vi "IMAQ FPGA Image Transfer to Target U32.vi"(6 "Image Transfer Size Alignment":u32(ring)=1 items=["1 Pixel"=1, "8 Pixels"=8], 7 "Write Timeout (ms)":i32=5000, 8 "error in (no error)":errorcluster, 9 "DMA FIFO Reference In":refnum<k20>, 10 "Maximum Pixels per Write":i32=-1, 11 "Image":T1) -> (0 "error out":errorcluster, 1 "DMA FIFO Reference Out":refnum<k20>, 3 "Image Out":T1)   [LabVIEW 2020, in "NI_VDM_FPGA_Basics.lvlib"]
doc: "Transfers an image from the host processor to the target FPGA via a DMA FIFO."
uses:
  <vilib>/visionFPGA/NI_VDM_FPGA_Basics.lvlib
  <vilib>/vision/Image Controls.llb/IMAQ Image.ctl
  <vilib>/rvi/errors/niLvFpgaAdjustHostInterfaceError.vi
  <vilib>/rvi/interface/nirviMethod/nirviMethod.xnode
  <vilib>/rvi/errors/niLvFpgaMergeErrorWithErrorCode.vi
  nivissvc.dll
  <vilib>/FPGAPlugInAG/Dynamic/niLvFpga_AcquireWriteRegionFifo_Dynamic.vi
  <vilib>/FPGAPlugInAG/Dynamic/niLvFpga_WriteFifo_Dynamic.vi
  <vilib>/vision/EDVR.llb/IMAQ ImageToEDVR 2D U32.vi
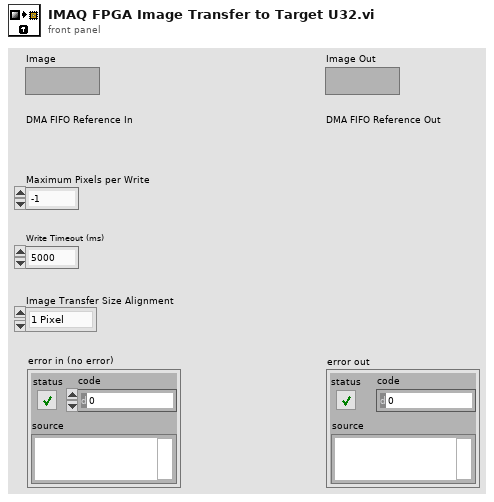
[diagram p1: front panel]
types:
  T1 = typedef "IMAQ Image.ctl" = refnum<image>
  T2 = typedef "Image Type" = u32
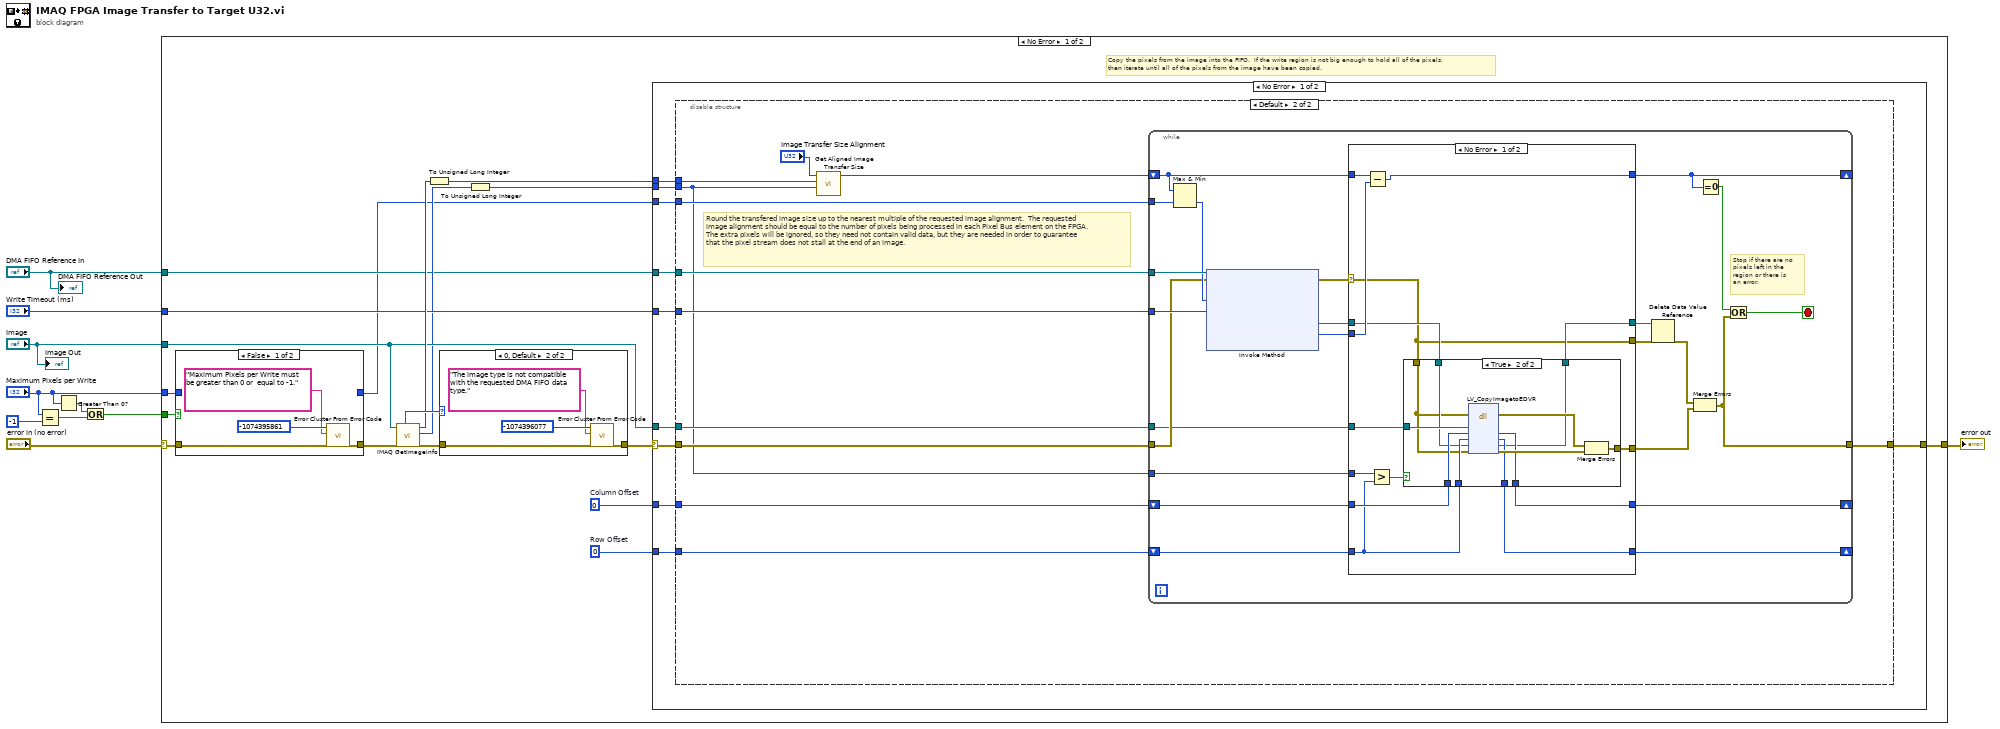
[diagram p0: block diagram]
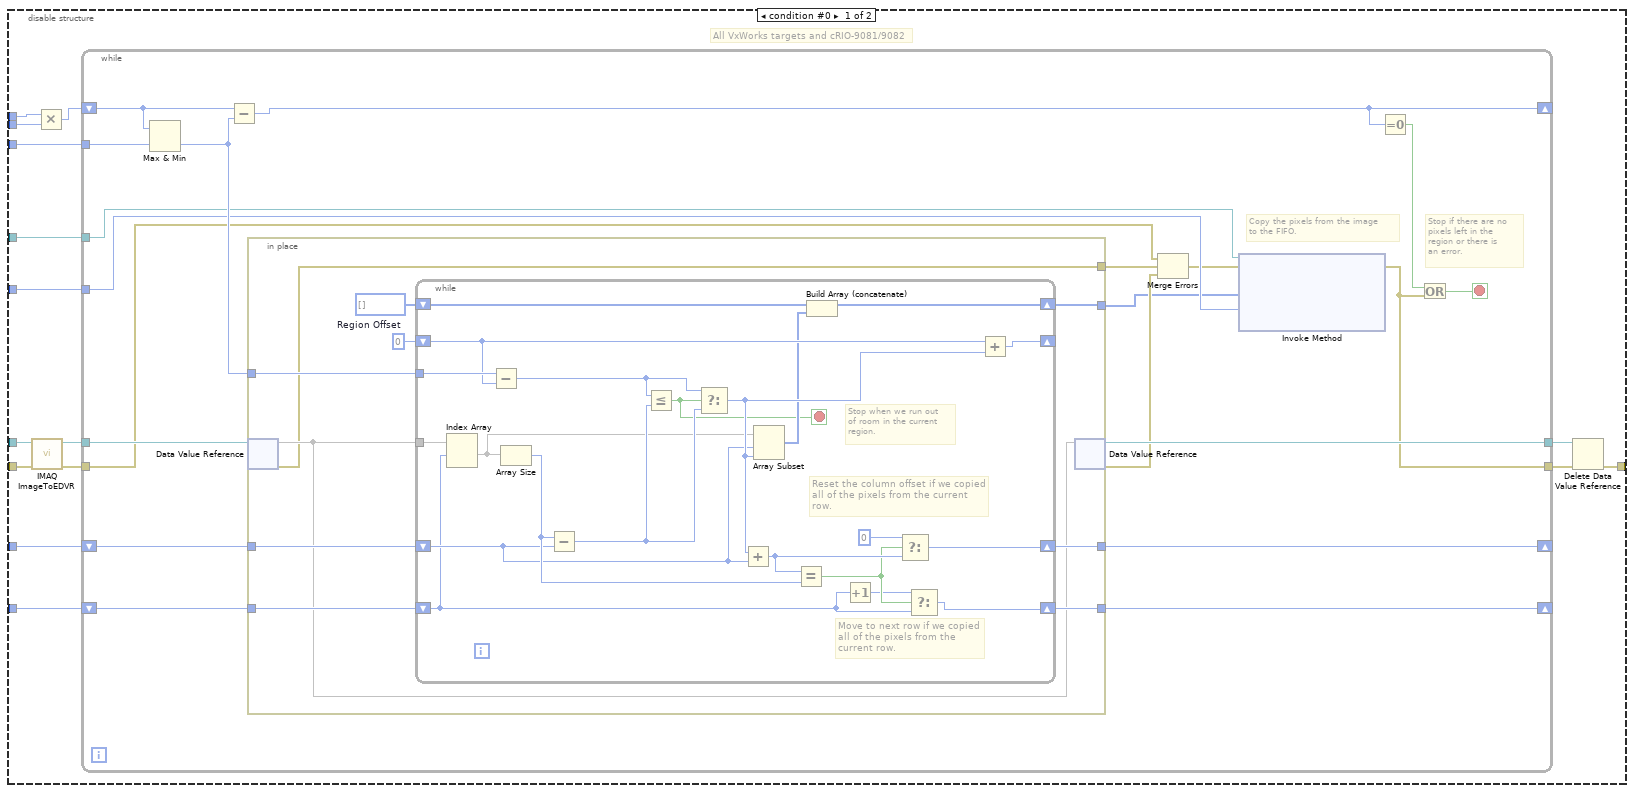
[diagram p2: hidden frame]
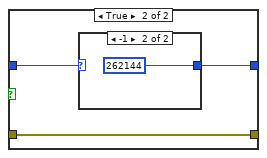
[diagram p6: hidden frame]
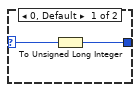
[diagram p7: hidden frame]
diagram:
  n1 = Equal?(x="Maximum Pixels per Write", y=-1) -> (x = y?=w6:bool)
  n2 = Greater Than 0?(x="Maximum Pixels per Write") -> (x > 0?=w7:bool)
  n3 = Or(x=w7, y=w6) -> (x .or. y?=w5:bool)
  n4 = case shown="No Error" "error in (no error)" {
    selector: "error in (no error)" -> [w23 w190]
    tunnel: "DMA FIFO Reference In" -> [w14 _]
    tunnel: "Write Timeout (ms)" -> [w16 _]
    tunnel: w5 -> [w26 _]
    tunnel: "Maximum Pixels per Write" -> [w24 _]
    tunnel: "Image" -> [w18 _]
    tunnel: [w21 w190] -> w2
    frame No Error {
      w20 = u32 0  # Row Offset
      w19 = u32 0  # Column Offset
      # "Copy the pixels from the image into the FIFO.  If the write region is not big enough to hold all of the pixels,\nthen iterate until all of the pixels from the image have been copied."
      n5 = case shown="False" w26 {
        tunnel: w23 -> [w176 w181]
        tunnel: [w175 w181] -> w25
        tunnel: w24 -> [_ w180]
        tunnel: [_ w179] -> w13
        frame False {
          n6 = call <vilib>:"Error Cluster From Error Code.vi"("error in (no error)"=w176, "error message (\"\")"="Maximum Pixels per Write must be greater than 0 or  equal to -1." ("error message (\"\")"), "error code (0)"=-1074395861) -> ("error out"=w175:errorcluster)  [unwired: 6 in]
        }
        frame True {
          n7 = case shown="-1" w180 {
            selector: w180 -> [w183 _]
            tunnel: [w182 u32 262144 ("Maximum Pixels per Write")] -> w179
            frame 0, Default {
              n8 = To Unsigned Long Integer(number=w183) -> (unsigned 32bit integer=w182:u32)
            }
            frame -1 {
            }
          }
        }
      }
      n9 = call "IMAQ GetImageInfo"("error in (no error)"=w25, "Image"=w18) -> ("error out"=w27:errorcluster, "Y Resolution"=w15:i32, "X Resolution"=w22:i32, "Image Type"=w28:T2)  [unwired: 2 in, 4 out]
      n10 = To Unsigned Long Integer(number=w22) -> (unsigned 32bit integer=w12:u32)
      n11 = case shown="0, Default" w28 {
        tunnel: w27 -> [w185 w187]
        tunnel: [w185 w186] -> w17
        frame 4, 5 {
          # "Allowed types are:\nRGB (U32)\nHSL (U32)"
        }
        frame 0, Default {
          n12 = call <vilib>:"Error Cluster From Error Code.vi"("error in (no error)"=w187, "error message (\"\")"="The image type is not compatible with the requested DMA FIFO data type." ("error message (\"\")"), "error code (0)"=-1074396077) -> ("error out"=w186:errorcluster)  [unwired: 6 in]
        }
      }
      n13 = To Unsigned Long Integer(number=w15) -> (unsigned 32bit integer=w11:u32)
      n14 = case shown="No Error" w17 {
        selector: w17 -> [w33 w174]
        tunnel: w19 -> [w35 _]
        tunnel: w20 -> [w34 _]
        tunnel: w14 -> [w37 _]
        tunnel: [w31 w174] -> w21
        tunnel: w13 -> [w38 _]
        tunnel: w16 -> [w36 _]
        tunnel: w18 -> [w32 _]
        tunnel: w12 -> [w30 _]
        tunnel: w11 -> [w29 _]
        frame No Error {
          n15 = disable-structure shown="Default" {
            disable-tunnel: w35 -> [w53 w116]
            disable-tunnel: w34 -> [w52 w115]
            disable-tunnel: w37 -> [w51 w114]
            disable-tunnel: [w42 w113] -> w31
            disable-tunnel: w38 -> [w50 w112]
            disable-tunnel: w36 -> [w49 w111]
            disable-tunnel: w33 -> [w47 w110]
            disable-tunnel: w32 -> [w48 w109]
            disable-tunnel: w30 -> [w40 w106]
            disable-tunnel: w29 -> [w41 w105]
            frame condition #0 {
              # "All VxWorks targets and cRIO-9081/9082"
              n16 = call-poly <vilib>:"IMAQ ImageToEDVR.vi"("error out"=w47, "Image"=w48) -> ("error out"=w45:errorcluster, "EDVR 2D U32"=w46:refnum<data-value>)  [unwired: 7 in, 1 out]
              n17 = Multiply(x=w40, y=w41) -> (x*y=w39:u32)
              n18 = while {
                shift-right: [w67] -> _
                shift-left: w39 -> [w64]
                tunnel: w46 -> [w73]
                shift-right: [w69] -> _
                shift-left: w53 -> [w71]
                shift-right: [w72] -> _
                shift-left: w52 -> [w70]
                tunnel: w51 -> [w58]
                tunnel: [w68] -> w44
                tunnel: [w56] -> w43
                tunnel: w50 -> [w63]
                tunnel: w49 -> [w59]
                tunnel: w45 -> [w54]
                stop <- w66 stop-if-true
                # "Copy the pixels from the image\nto the FIFO."
                # "Stop if there are no\npixels left in the \nregion or there is\nan error."
                n19 = Max & Min(x=w64, y=w63) -> (min(x,y)=w62:u32)  [unwired: 1 out]
                n20 = Subtract(x=w64, y=w62) -> (x-y=w67:u32)
                n21 = in-place {
                  in-place-border: w62 -> [w81]
                  in-place-border: [w83] -> w72
                  in-place-border: w71 -> [w80]
                  in-place-border: w70 -> [w78]
                  in-place-border: [w79] -> w69
                  in-place-border: [w75] -> w61
                  in-place-border: [w74] -> w55
                  w82 = u32 0  # Region Offset
                  n22 = in-place-dvr #1(w73) -> (w77:u32[][], w75:errorcluster)
                  n23 = while {
                    tunnel: w77 -> [w90]
                    shift-right: [w102] -> _
                    shift-left: w82 -> [w101]
                    tunnel: w81 -> [w104]
                    shift-right: [w95] -> w79
                    shift-left: w80 -> [w91]
                    shift-right: [w85] -> w74
                    shift-left: u8[] [] -> [w87]
                    shift-right: [w92] -> w83
                    shift-left: w78 -> [w88]
                    stop <- w84 stop-if-true
                    # "Stop when we run out\nof room in the current\nregion."
                    # "Reset the column offset if we copied\nall of the pixels from the current\nrow."
                    # "Move to next row if we copied\nall of the pixels from the\ncurrent row."
                    n24 = Index Array(array=w90, index (row)=w88) -> (element=w89:u32[])  [unwired: 1 in]
                    n25 = Subtract(x=w104, y=w101) -> (x-y=w103:u32)
                    n26 = Array Size(array=w89) -> (size(s)=w100:i32)
                    n27 = Subtract(x=w100, y=w91) -> (x-y=w98:u32)
                    n28 = Less Or Equal?(x=w103, y=w98) -> (x <= y?=w84:bool)
                    n29 = Select(t=w103, s=w84, f=w98) -> (s? t:f=w99:u32)
                    n30 = Add(x=w99, y=w91) -> (x+y=w96:u32)
                    n31 = Array Subset(array=w89, index=w91, length=w99) -> (w86:u32[])
                    n32 = Equal?(x=w96, y=w100) -> (x = y?=w94:bool)
                    n33 = Build Array (concatenate)(w87, w86) -> (w85:u32[])
                    n34 = Increment(x=w88) -> (x+1=w93:u32)
                    n35 = Select(t=u32 0 ("Elements In Region"), s=w94, f=w96) -> (s? t:f=w95:u32)
                    n36 = Select(t=w93, s=w94, f=w88) -> (s? t:f=w92:u32)
                    n37 = Add(x=w101, y=w99) -> (x+y=w102:u32)
                  }
                  n38 = in-place-dvr #1(w77) -> (w68:refnum<data-value>, w60:errorcluster)
                }
                n39 = Merge Errors(w54, w61, w60) -> (w57:errorcluster)
                n40 = xnode "Invoke Method"("FPGA VI Reference In"=w58, "error in"=w57, "Data"=w55, "Timeout (ms)"=w59) -> ("error out"=w56:errorcluster)  [unwired: 2 out]
                n41 = Equal To 0?(x=w67) -> (x = 0?=w65:bool)
                n42 = Or(x=w65, y=w56) -> (x .or. y?=w66:bool)
              }
              n43 = Delete Data Value Reference(data value reference=w44, error in=w43) -> (error out=w42:errorcluster)  [unwired: 1 out]
            }
            frame condition #1 (active) {
              # "Round the transfered image size up to the nearest multiple of the requested image alignment.  The requested image alignment should be equal to the number of pixels being processed in each Pixel Bus element on the FPGA.The extra pixels will be ignored, so they need not contain valid data, but they are needed in order to guarantee that the pixel stream does not stall at the end of an image."
              n44 = call <vilib>:"Get Aligned Image Transfer Size.vi"("Y Resolution"=w105, "X Resolution"=w106, "Image Transfer Size Alignment"="Image Transfer Size Alignment") -> ("Aligned Image Transfer Size"=w107:u64)  [unwired: 8 in]
              n45 = while {
                shift-right: [w127] -> _
                shift-left: w107 -> [w122]
                shift-right: [w134] -> _
                shift-left: w116 -> [w136]
                shift-right: [w137] -> _
                shift-left: w115 -> [w135]
                tunnel: w114 -> [w133]
                tunnel: [w125] -> w113
                tunnel: w112 -> [w121]
                tunnel: w111 -> [w120]
                tunnel: w110 -> [w119]
                tunnel: w109 -> [w118]
                tunnel: w105 -> [w117]
                stop <- w126 stop-if-true
                # "Stop if there are no\npixels left in the \nregion or there is\nan error."
                n46 = Max & Min(x=w122, y=w121) -> (min(x,y)=w123:u64)  [unwired: 1 out]
                n47 = xnode "Invoke Method"("FPGA VI Reference In"=w133, "error in"=w119, "Number of Elements"=w123, "Timeout (ms)"=w120) -> ("error out"=w132:errorcluster, "Write Region Reference"=w139:refnum<data-value>, "Elements In Region"=w138:u32)  [unwired: 2 out]
                n48 = case shown="No Error" w132 {
                  selector: w132 -> [w143 w170]
                  tunnel: w122 -> [w153 w173]
                  tunnel: [w152 w173] -> w127
                  tunnel: w139 -> [w148 w169]
                  tunnel: w138 -> [w151 _]
                  tunnel: [w145 w171] -> w137
                  tunnel: w136 -> [w149 w172]
                  tunnel: w135 -> [w141 w171]
                  tunnel: [w146 w172] -> w134
                  tunnel: [w144 w169] -> w131
                  tunnel: [w143 w170] -> w130
                  tunnel: [w147 _] -> w128
                  tunnel: w118 -> [w150 _]
                  tunnel: w117 -> [w140 _]
                  frame No Error {
                    n49 = Subtract(x=w153, y=w151) -> (x-y=w152:u64)
                    n50 = Greater?(x=w140, y=w141) -> (0:w142:bool)
                    n51 = case shown="True" w142 {
                      tunnel: w150 -> [_ w168]
                      tunnel: w149 -> [w154 w167]
                      tunnel: w141 -> [w155 w166]
                      tunnel: w148 -> [w156 w164]
                      tunnel: [w157 w162] -> w147
                      tunnel: [w154 w161] -> w146
                      tunnel: [w155 w160] -> w145
                      tunnel: [w156 w159] -> w144
                      tunnel: w143 -> [w157 w158]
                      frame False {
                      }
                      frame True {
                        n52 = dll-call lib="nivissvc.*" fn="LV_CopyImagetoEDVR" label="LV_CopyImageToEDVR"(error in=w158, "image"=w168, "xImageOffset"=w167, "yImageOffset"=w166, "EDVR"=w164, "error"=w158) -> (error out=w165:errorcluster, "xImageOffset"=w161:u32, "yImageOffset"=w160:u32, "EDVR"=w159:refnum<data-value>, "error"=w163:errorcluster)  [unwired: 4 in, 1 out]
                        n53 = Merge Errors(w165, w163) -> (w162:errorcluster)
                      }
                    }
                  }
                  frame Error {
                  }
                }
                n54 = Delete Data Value Reference(data value reference=w131, error in=w130) -> (error out=w129:errorcluster)  [unwired: 1 out]
                n55 = Merge Errors(w129, w128) -> (w125:errorcluster)
                n56 = Equal To 0?(x=w127) -> (x = 0?=w124:bool)
                n57 = Or(x=w124, y=w125) -> (x .or. y?=w126:bool)
              }
            }
          }
        }
        frame Error {
        }
      }
    }
    frame Error {
    }
  }
  "error out" <- w2
  "Image Out" <- "Image"
  "DMA FIFO Reference Out" <- "DMA FIFO Reference In"
